vi "Rotate.vi"(9 "Theta (Radians)":dbl=1.57, 10 "Pivot Point":cluster{"X":dbl, "Y":dbl}={"X"=1.0, "Y"=1.0}, 11 "Points to Rotate":cluster{dbl, dbl}[](array[cluster])=[{2.0, 2.0}, {3.0, 3.0}, {4.0, 4.0}]) -> (3 "Rotated Points":cluster{"x out":dbl, "y out":dbl}[](array[cluster]))   [LabVIEW 2016]
uses:
  <vilib>/Analysis/coordinate.llb/2D Cartesian Coordinate Shift (Scalar).vi
  <vilib>/Analysis/coordinate.llb/2D Cartesian Coordinate Rotation (Scalar).vi
  <vilib>/Analysis/NI_AALPro.lvlib
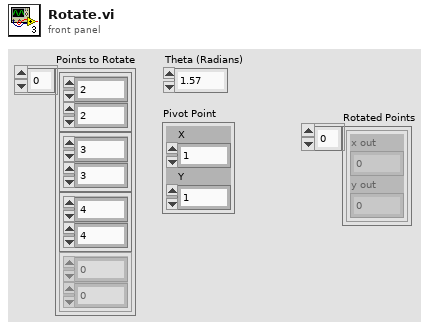
[diagram p1: front panel]
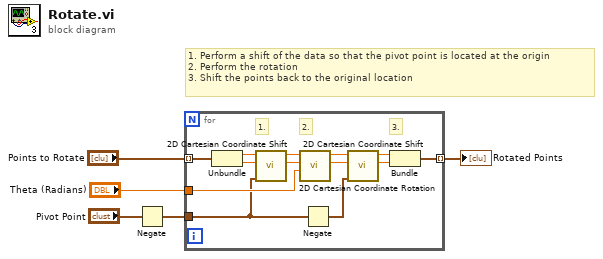
[diagram p0: block diagram]
diagram:
  # "1. Perform a shift of the data so that the pivot point is located at the origin\n2. Perform the rotation\n3. Shift the points back to the original location"
  n1 = Negate(x="Pivot Point") -> (-x=w4:cluster{"X":dbl, "Y":dbl})
  n2 = for {
    tunnel: "Points to Rotate" -> [w18] mode=indexing
    tunnel: w4 -> [w16]
    tunnel: "Theta (Radians)" -> [w17]
    tunnel: [w13] -> w1 mode=indexing
    # "3."
    # "2."
    # "1."
    n3 = Unbundle(w18) -> (w12:dbl, w11:dbl)
    n4 = call-poly <vilib>:"2D Cartesian Coordinate Shift.vi"("shift"=w16, "y"=w11, "x"=w12) -> ("y out"=w7:dbl, "x out"=w8:dbl)  [unwired: 6 in, 1 out]
    n5 = call-poly <vilib>:"2D Cartesian Coordinate Rotation.vi"("theta"=w17, "y"=w7, "x"=w8) -> ("y out"=w9:dbl, "x out"=w10:dbl)  [unwired: 6 in, 1 out]
    n6 = Negate(x=w16) -> (-x=w6:cluster{"X":dbl, "Y":dbl})
    n7 = call-poly <vilib>:"2D Cartesian Coordinate Shift.vi"("shift"=w6, "y"=w9, "x"=w10) -> ("y out"=w14:dbl, "x out"=w15:dbl)  [unwired: 6 in, 1 out]
    n8 = Bundle("x out"=w15, "y out"=w14) -> (w13:cluster{"x out":dbl, "y out":dbl})  [unwired: 1 in]
  }
  "Rotated Points" <- w1
